vi "Module Top Level.vi"(8 "error in":errorcluster, 11 "FPGA Ref":T1) -> (0 "error out":errorcluster)   [LabVIEW 2018, in "Vibration.lvlib"]
doc: "This is the top level VI for this module. It uses a queue for communications and is stopped user a user event. The general architecture is similar to a simple queued message handler.\n\nThe VIs associated with this module are organized in a LabVIEW Library."
uses:
  Vibration.lvlib
  FPGA/FPGA VI Reference.ctl
  Private Controls/Host Comms Data.ctl
  Modules/Testing UI 3/Private Controls/Cutoff Frequency.ctl
  Private Controls/Module Data.ctl
  Private Controls/Module Action.ctl
  <vilib>/LabVIEW Targets/FPGA/cRIO/shared/nicrio_ModuleControls/nicrio_cRIO-9234_ConfigModeRing.ctl
  <vilib>/LabVIEW Targets/FPGA/cRIO/shared/nicrio_ModuleControls/nicrio_cRIO-9234_DataRatesRing2.ctl
  <vilib>/rvi/interface/common/niFpgaWaitOnOcc.vi
  <vilib>/Utility/error.llb/Error Cluster From Error Code.vi
  <vilib>/rvi/errors/niLvFpgaAdjustHostInterfaceError.vi
  <vilib>/rvi/interface/nirviMethod/nirviMethod.xnode
  <vilib>/rvi/interface/nirviReadWriteControl/nirviReadWriteControl.xnode
  <vilib>/rvi/errors/niLvFpgaMergeErrorWithErrorCode.vi
  <vilib>/FPGAPlugInAG/Dynamic/niLvFpga_AcknowledgeIrq_Dynamic.vi
  Modules/Testing UI 3/Testing UI 3.lvlib
  <vilib>/FPGAPlugInAG/Dynamic/niLvFpga_ConfigureFifo_Dynamic.vi
  <vilib>/FPGAPlugInAG/Dynamic/niLvFpga_StartFifo_Dynamic.vi
  NiFpgaLv.dll
  <vilib>/rvi/interface/Simulation/niFpgaSimulationCallBeginRW.vi
panel:
  # "Vibration"
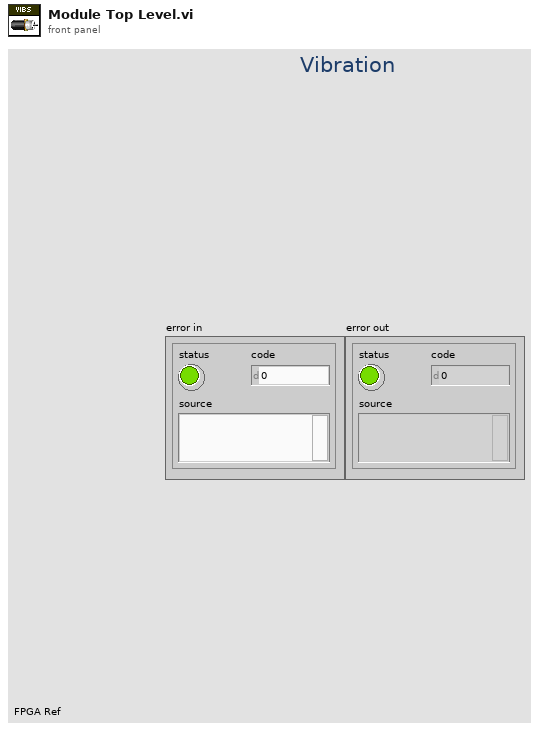
[diagram p1: front panel]
types:
  T1 = typedef "FPGA VI Reference.ctl" = refnum<k20>
  T2 = typedef "Vibration.lvlib/Host Comms Data.ctl" = cluster{"FPGARef":T1, "Data Rate(Hz)":dbl, "Sensitivities(mv/(m/s2))":dbl[], "Cutoff Frequncies":T3[], "Waterfall Select":u8}
  T3 = typedef "Testing UI 3.lvlib/Cutoff Frequency.ctl" = cluster{"LP Passband":dbl, "HP Stopband":dbl, "LP Stopband":dbl, "HP Passband":dbl}
  T4 = typedef "Vibration.lvlib/Module Data.ctl" = cluster{"Data":variant, "Action":T5}
  T5 = typedef "Vibration.lvlib/Module Action.ctl" = enum16{"Init", "Waterfall Select", "Read", "Accel Sensitivities", "Filters", "Error"}
  T6 = typedef "nicrio_cRIO-9234_DataRatesRing2.ctl" = u8
  T7 = typedef "nicrio_cRIO-9234_ConfigModeRing.ctl" = u8
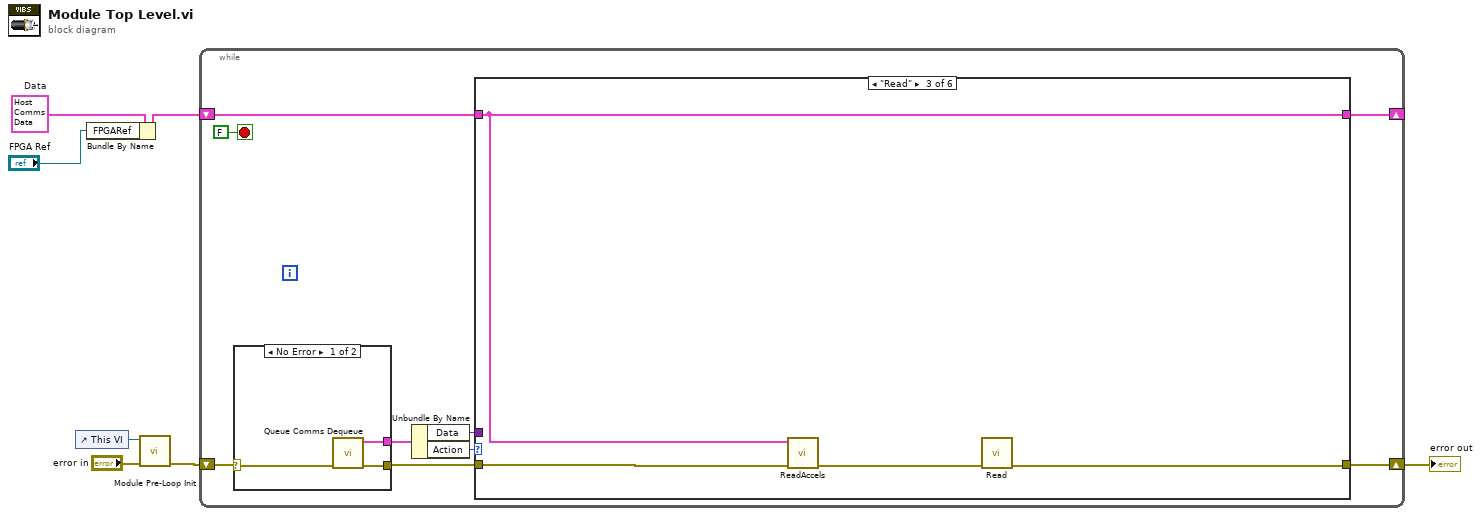
[diagram p0: block diagram]
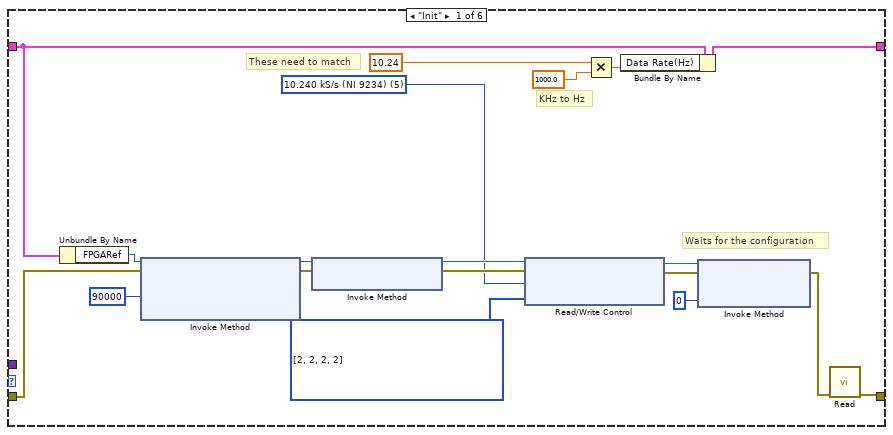
[diagram p2: hidden frame]
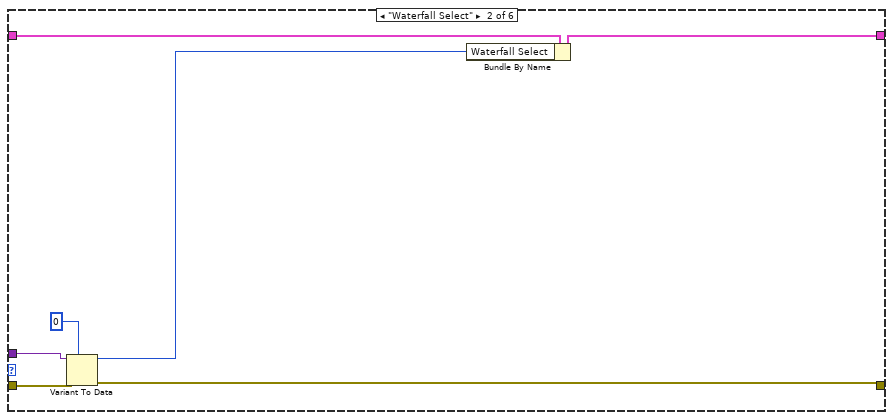
[diagram p3: hidden frame]
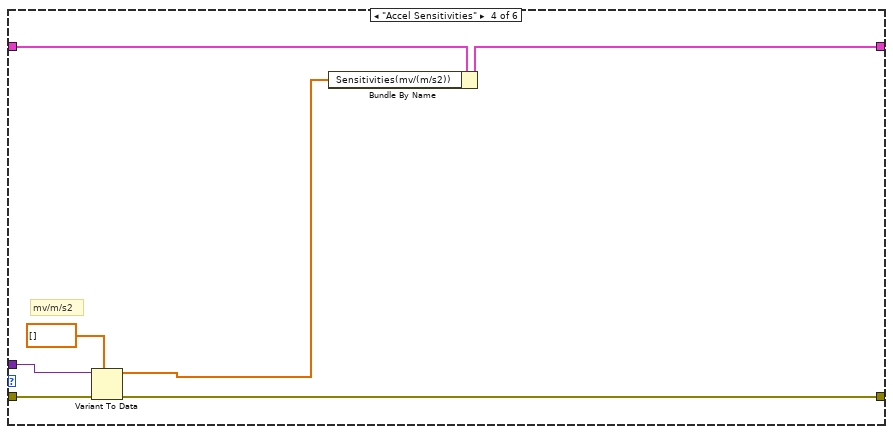
[diagram p4: hidden frame]
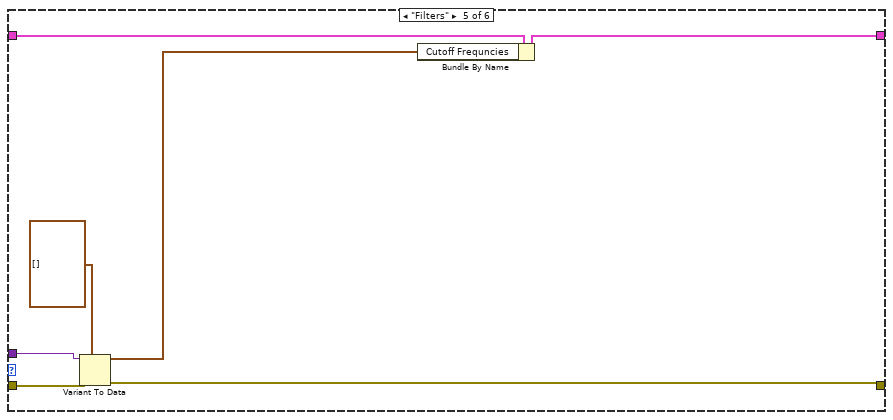
[diagram p5: hidden frame]
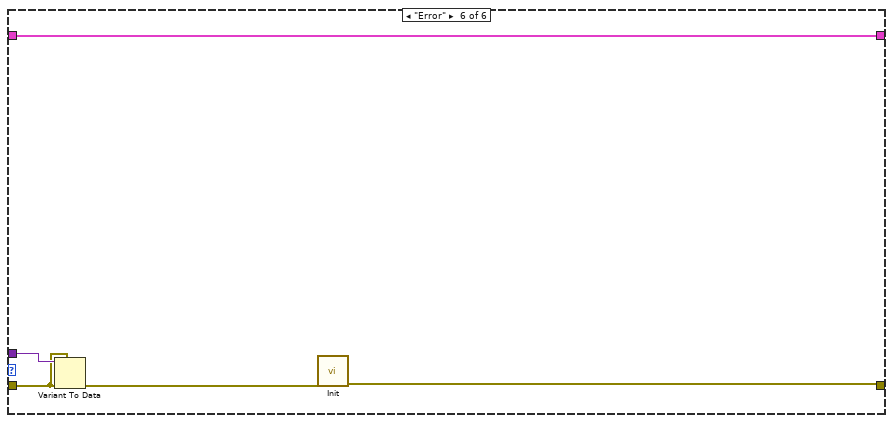
[diagram p6: hidden frame]
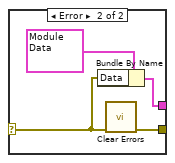
[diagram p7: hidden frame]
diagram:
  w4 = T2 {"FPGARef"=refnum, "Data Rate(Hz)"=0.0, "Sensitivities(mv/(m/s2))"=[0.0, 0.0, 0.0, 0.0], "Cutoff Frequncies"=[], "Waterfall Select"=0}  # Data
  n1 = control-ref of="This VI"() -> (w7:refnum<vi>)
  n2 = Bundle By Name(cluster=w4, "FPGARef"="FPGA Ref") -> (w2:T2)
  n3 = call "Module Pre-Loop Init.vi"("error in (no error)"="error in", "Top Level VI Ref in"=w7) -> ("error out"=w3:errorcluster)  [unwired: 9 in]
  n4 = while {
    shift-right: [w12] -> w5
    shift-left: w3 -> [w11]
    shift-right: [w10] -> _
    shift-left: w2 -> [w9]
    stop <- FALSE stop-if-true
    n5 = case shown="No Error" w11 {
      selector: w11 -> [w67 w70]
      tunnel: [w68 w71] -> w16
      tunnel: [w66 w69] -> w13
      frame No Error {
        n6 = call "Queue Comms Dequeue.vi"("error in (no error)"=w67) -> ("error out"=w66:errorcluster, "element"=w68:T4)  [unwired: 9 in]
      }
      frame Error {
        n7 = Bundle By Name(cluster=T4 {"Data"=variant, "Action"=enum."Error"} ("element"), "Data"=w70) -> (w71:T4)
        n8 = call <vilib>:"Clear Errors.vi"("error in (no error)"=w70) -> ("error out"=w69:errorcluster)  [unwired: 5 in, 1 out]
      }
    }
    n9 = Unbundle By Name(w16) -> ("Data"=w14:variant, "Action"=w15:T5)
    n10 = case shown="\"Read\"" w15 {
      tunnel: w14 -> [_ w40 _ w50 w58 w65]
      tunnel: w13 -> [w24 w41 w45 w52 w59 w64]
      tunnel: [w22 w38 w43 w51 w54 w62] -> w12
      tunnel: [w21 w37 w46 w48 w56 w61] -> w10
      tunnel: w9 -> [w26 w42 w46 w53 w60 w61]
      frame "Init" {
        w17 = T6 5 items=["51.200 kS/s (NI 9234)"=1, "25.600 kS/s (NI 9234)"=2, "17.067 kS/s (NI 9234)"=3, "12.800 kS/s (NI 9234)"=4, "10.240 kS/s (NI 9234)"=5, "8.533 kS/s (NI 9234)"=6, "7.314 kS/s (NI 9234)"=7, "6.400 kS/s (NI 9234)"=8, "5.689 kS/s (NI 9234)"=9, "5.120 kS/s (NI 9234)"=10, "4.654 kS/s (NI 9234)"=11, "4.267 kS/s (NI 9234)"=12, "3.938 kS/s (NI 9234)"=13, "3.657 kS/s (NI 9234)"=14, "3.413 kS/s (NI 9234)"=15, "3.200 kS/s (NI 9234)"=16, "3.012 kS/s (NI 9234)"=17, "2.845 kS/s (NI 9234)"=18, "2.695 kS/s (NI 9234)"=19, "2.560 kS/s (NI 9234)"=20, "2.438 kS/s (NI 9234)"=21, "2.328 kS/s (NI 9234)"=22, "2.226 kS/s (NI 9234)"=23, "2.133 kS/s (NI 9234)"=24, "2.048 kS/s (NI 9234)"=25, "1.969 kS/s (NI 9234)"=26, "1.896 kS/s (NI 9234)"=27, "1.829 kS/s (NI 9234)"=28, "1.765 kS/s (NI 9234)"=29, "1.707 kS/s (NI 9234)"=30, "1.652 kS/s (NI 9234)"=31] ("Data Rate")
        w29 = T7[] [2, 2, 2, 2] items=["AC Coupled", "DC Coupled", "IEPE AC Coupled"] ("Accelerometer Configs")
        # "Waits for the configuration"
        # "KHz to Hz"
        # "These need to match"
        n11 = Unbundle By Name(w26) -> ("FPGARef"=w25:T1)
        n12 = xnode "Invoke Method"("FPGA VI Reference In"=w25, "error in"=w24, "Requested Depth"=u32 90000 ("FPGA FIFO Buffer Size")) -> ("FPGA VI Reference Out"=w33:T1, "error out"=w32:errorcluster)  [unwired: 1 out]
        n13 = xnode "Invoke Method"("FPGA VI Reference In"=w33, "error in"=w32) -> ("FPGA VI Reference Out"=w31:T1, "error out"=w30:errorcluster)
        n14 = xnode "Read/Write Control"("FPGA VI Reference In"=w31, "error in"=w30, "Data Rate"=w17, "Accelerometer Configs"=w29) -> ("FPGA VI Reference Out"=w34:T1, "error out"=w35:errorcluster)
        n15 = Multiply(x=10.24 ("Data Rate(KHz)"), y=1000.0 ("x")) -> (x*y=w18:dbl)
        n16 = Bundle By Name(cluster=w26, "Data Rate(Hz)"=w18) -> (w21:T2)
        n17 = xnode "Invoke Method"("FPGA VI Reference In"=w34, "error in"=w35, "IRQ Number(s)"=0) -> ("error out"=w23:errorcluster)  [unwired: 1 out]
        n18 = call "Read.vi"("error in"=w23) -> ("error out"=w22:errorcluster)  [unwired: 10 in]
      }
      frame "Waterfall Select" {
        n19 = Variant To Data(error in=w41, type=u8 0, Variant=w40) -> (data=w36:u8, error out=w38:errorcluster)
        n20 = Bundle By Name(cluster=w42, "Waterfall Select"=w36) -> (w37:T2)
      }
      frame "Read" {
        n21 = call "ReadAccels.vi"("error in"=w45, "Data"=w46) -> ("error out"=w44:errorcluster)  [unwired: 9 in]
        n22 = call "Read.vi"("error in"=w44) -> ("error out"=w43:errorcluster)  [unwired: 10 in]
      }
      frame "Accel Sensitivities" {
        # "mv/m/s2"
        n23 = Variant To Data(error in=w52, type=dbl[] [] ("Accel Sensistivity"), Variant=w50) -> (data=w47:dbl[], error out=w51:errorcluster)
        n24 = Bundle By Name(cluster=w53, "Sensitivities(mv/(m/s2))"=w47) -> (w48:T2)
      }
      frame "Filters" {
        n25 = Variant To Data(error in=w59, type=T3[] [] ("Cutoff Frequncies"), Variant=w58) -> (data=w55:T3[], error out=w54:errorcluster)
        n26 = Bundle By Name(cluster=w60, "Cutoff Frequncies"=w55) -> (w56:T2)
      }
      frame "Error" {
        n27 = Variant To Data(error in=w64, type=w64, Variant=w65) -> (error out=w63:errorcluster)  [unwired: 1 out]
        n28 = call "Init.vi"("error in"=w63) -> ("error out"=w62:errorcluster)  [unwired: 10 in]
      }
    }
  }
  "error out" <- w5
